vi "HelloWorld.vi"(8 "数值 2":dbl, 11 "数值":dbl) -> (3 "数值 3":dbl)   [LabVIEW 2017]
panel:
  in  "停止":bool
  out "字符串":string
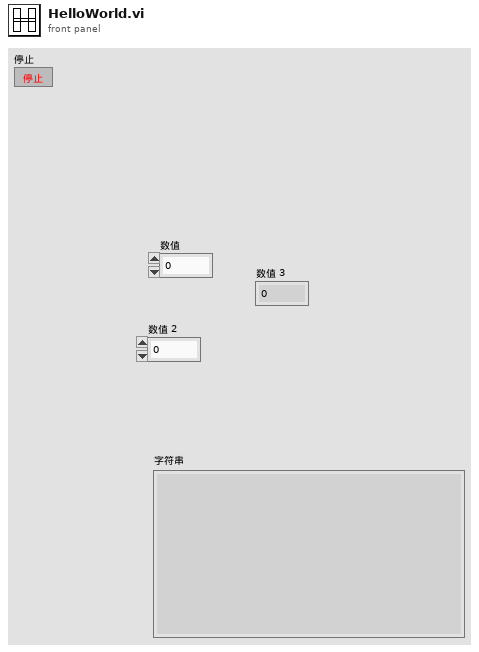
[diagram p1: front panel]
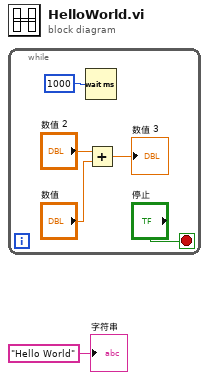
[diagram p0: block diagram]
diagram:
  n1 = while {
    stop <- "停止" stop-if-true
    n2 = Wait (ms)(milliseconds to wait=u32 1000 ("等待时间（毫秒）")) -> ()  [unwired: 1 out]
    n3 = Add(x="数值 2", y="数值") -> (x+y=→"数值 3":dbl)
  }
  "字符串" <- "Hello World"
